vi "INTERFAZ.vi"() -> ()   [LabVIEW 2023]
uses:
  <vilib>/Instr/_visa.llb/VISA Configure Serial Port (Instr).vi
panel:
  in  "stop":bool
  in  "Tab Control":T1(tab)
  in  "PUERTO COM":refnum<visa-resource-name>
  out "TRAMA DE DATOS":string
  out "DATA SENSOR":string
  out "DATOS DE LOS SENSORES":string[](array[string])
  out "TERMOMETRO":dbl(slide) scale=0.0..150.0
  out "VOLTAJE":dbl(knob) scale=0.0..5.0
  out "DISTANCIA":dbl(slide) scale=0.0..100.0
  out "HUMEDAD":dbl(slide) scale=0.0..100.0
  out "LEDC":bool
  out "LEDB":bool
  out "STOP/RUN":bool
  out "RIGHT":bool
  out "LEFT":bool
  out "LEDA":bool
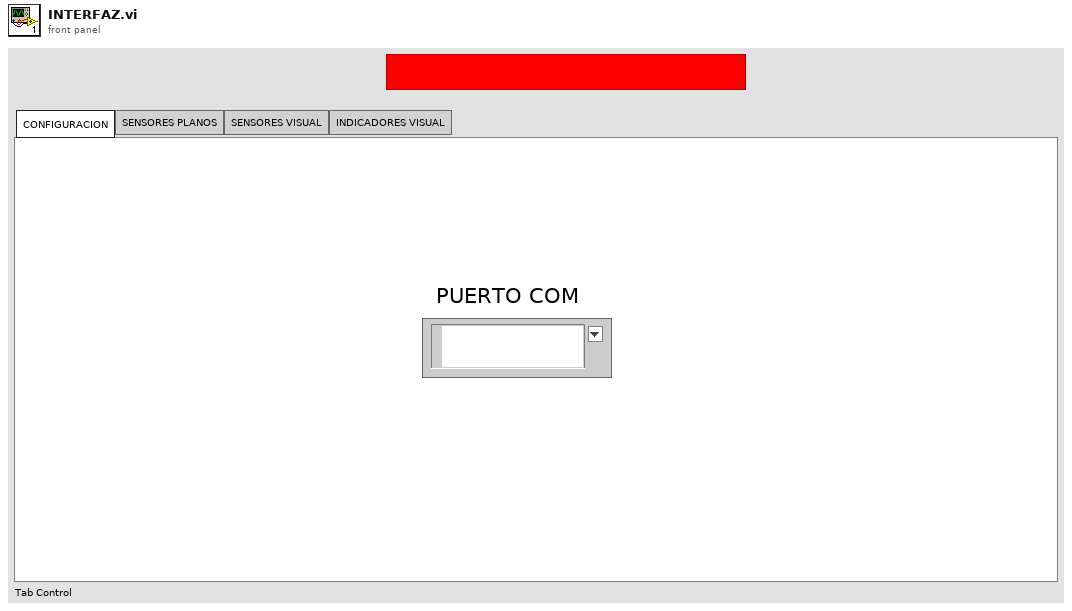
[diagram p1: front panel]
types:
  T1 = enum32{"CONFIGURACION", "SENSORES PLANOS", "SENSORES VISUAL", "INDICADORES VISUAL"}
  T2 = enum16{"ESPERAR DATA", "LEER DATA", "INTERPRETAR DATA ", "VISUALIZAR DATA"}
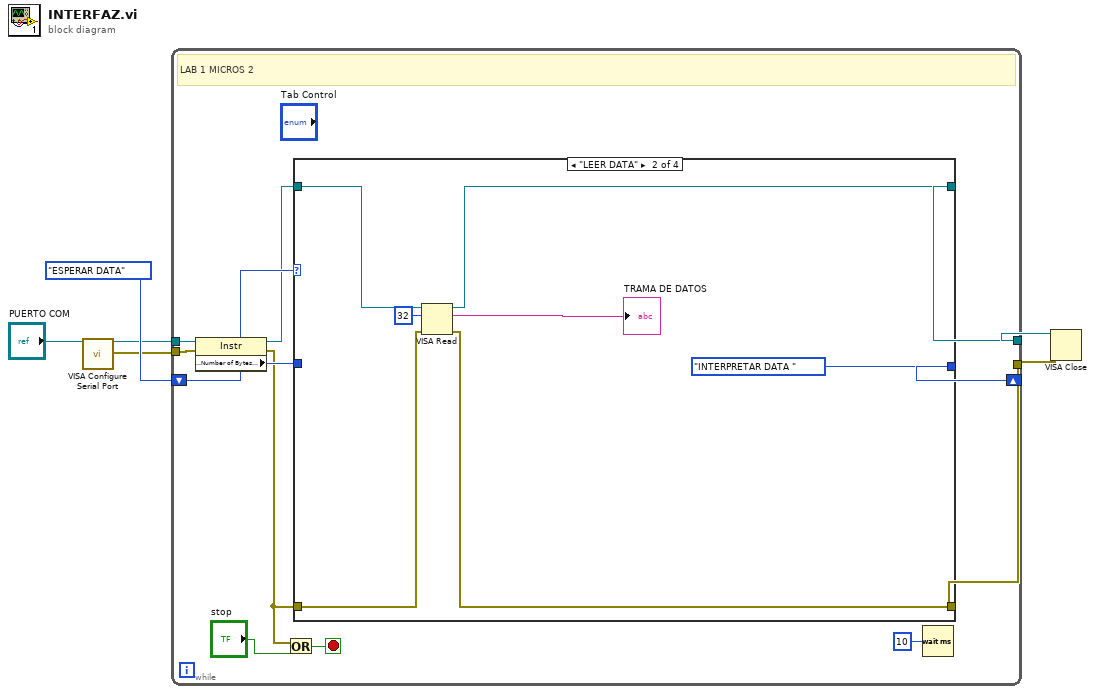
[diagram p0: block diagram]
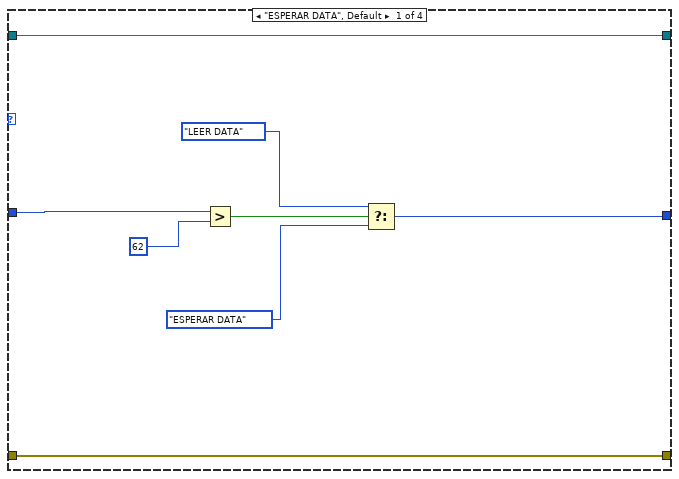
[diagram p2: hidden frame]
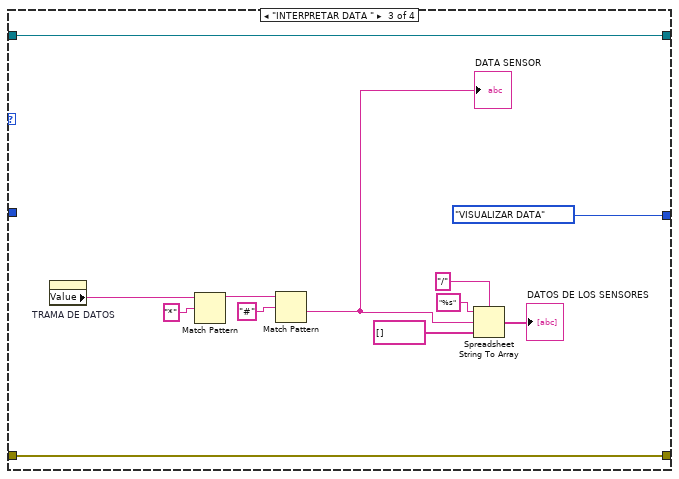
[diagram p3: hidden frame]
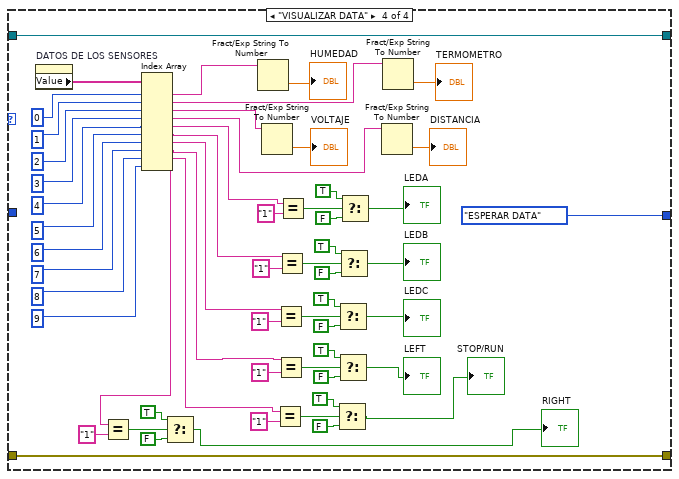
[diagram p4: hidden frame]
diagram:
  n1 = call-poly "VISA Configure Serial Port"("VISA resource name"="PUERTO COM") -> ("VISA resource name out"=w4:refnum<visa-resource-name>, "error out"=w3:errorcluster)  [unwired: 13 in]
  n2 = while {
    shift-right: [w14] -> _
    shift-left: T2."ESPERAR DATA" -> [w18]
    tunnel: w4 -> [w16]
    tunnel: w3 -> [w17]
    tunnel: [w12] -> w2
    tunnel: [w10] -> w1
    stop <- w9 stop-if-true
    # "LAB 1 MICROS 2"
    n3 = property class="Instr"(reference=w16, error in=w17) -> (reference out=w13:refnum<visa-resource-name>, error out=w7:errorcluster, "Serial Settings:Number of Bytes at Serial Port"=w15:u32)
    n4 = Or(x=w7, y="stop") -> (x .or. y?=w9:bool)
    n5 = case shown="\"LEER DATA\"" w18 {
      tunnel: w15 -> [w26 _ _ _]
      tunnel: [w21 T2."INTERPRETAR DATA " T2."VISUALIZAR DATA" T2."ESPERAR DATA"] -> w14
      tunnel: w13 -> [w20 w33 w44 w91]
      tunnel: [w20 w30 w44 w91] -> w12
      tunnel: w7 -> [w19 w29 w34 w49]
      tunnel: [w19 w28 w34 w49] -> w10
      frame "ESPERAR DATA", Default {
        n6 = Greater?(x=w26, y=u32 62) -> (0:w24:bool)
        n7 = Select(t=T2."LEER DATA", s=w24, f=T2."ESPERAR DATA") -> (s? t:f=w21:T2)
      }
      frame "LEER DATA" {
        n8 = VISA Read(VISA resource name=w33, byte count=u32 32, error in (no error)=w29) -> (VISA resource name out=w30:refnum<visa-resource-name>, read buffer=→"TRAMA DE DATOS":string, error out=w28:errorcluster)  [unwired: 1 out]
      }
      frame "INTERPRETAR DATA " {
        n9 = property on="TRAMA DE DATOS" class="Str"() -> ("Value"=w43:string)  [unwired: 2 in, 2 out]
        n10 = Match Pattern(string=w43, regular expression="*") -> (before substring=w41:string)  [unwired: 1 in, 3 out]
        n11 = Match Pattern(string=w41, regular expression="#") -> (after substring=w37:string)  [unwired: 1 in, 3 out]
        "DATA SENSOR" <- w37
        n12 = Spreadsheet String To Array(delimiter (Tab)="/", format string="%s", spreadsheet string=w37, array type (2D Dbl)=string[] []) -> (array=→"DATOS DE LOS SENSORES":string[])
      }
      frame "VISUALIZAR DATA" {
        n13 = property on="DATOS DE LOS SENSORES" class="Arr (strict)"() -> ("Value"=w102:string[])  [unwired: 2 in, 2 out]
        n14 = Index Array(array=w102, index #1=0 ("index"), index #2=1 ("index"), index #3=2 ("index"), index #4=3 ("index"), index #5=4 ("index"), index #6=5 ("index"), index #7=6 ("index"), index #8=7 ("index"), index #9=8 ("index"), index #10=9 ("index")) -> (element #1=w48:string, element #2=w47:string, element #3=w46:string, element #4=w88:string, element #5=w80:string, element #6=w79:string, element #7=w78:string, element #8=w52:string, element #9=w51:string, element #10=w50:string)
        n15 = Equal?(x=w50, y="1") -> (x = y?=w66:bool)
        n16 = Select(t=TRUE, s=w66, f=FALSE) -> (s? t:f=→"RIGHT":bool)
        n17 = Fract/Exp String To Number(string=w48) -> (number=→"HUMEDAD":dbl)  [unwired: 3 in, 1 out]
        n18 = Fract/Exp String To Number(string=w46) -> (number=→"VOLTAJE":dbl)  [unwired: 3 in, 1 out]
        n19 = Equal?(x=w51, y="1") -> (x = y?=w58:bool)
        n20 = Equal?(x=w78, y="1") -> (x = y?=w83:bool)
        n21 = Equal?(x=w52, y="1") -> (x = y?=w61:bool)
        n22 = Equal?(x=w79, y="1") -> (x = y?=w95:bool)
        n23 = Equal?(x=w80, y="1") -> (x = y?=w98:bool)
        n24 = Select(t=TRUE, s=w58, f=FALSE) -> (s? t:f=→"STOP/RUN":bool)
        n25 = Select(t=TRUE, s=w83, f=FALSE) -> (s? t:f=→"LEDC":bool)
        n26 = Select(t=TRUE, s=w61, f=FALSE) -> (s? t:f=→"LEFT":bool)
        n27 = Select(t=TRUE, s=w95, f=FALSE) -> (s? t:f=→"LEDB":bool)
        n28 = Select(t=TRUE, s=w98, f=FALSE) -> (s? t:f=→"LEDA":bool)
        n29 = Fract/Exp String To Number(string=w88) -> (number=→"DISTANCIA":dbl)  [unwired: 3 in, 1 out]
        n30 = Fract/Exp String To Number(string=w47) -> (number=→"TERMOMETRO":dbl)  [unwired: 3 in, 1 out]
      }
    }
    n31 = Wait (ms)(milliseconds to wait=u32 10) -> ()  [unwired: 1 out]
  }
  n32 = VISA Close(VISA resource name=w2, error in (no error)=w1) -> ()  [unwired: 1 out]
